vi "Setup Timer Parameters.vi"(7 "Timer Notifier":refnum<notifier>, 8 "error in (no error)":errorcluster, 9 "Count":i32, 10 "Period":i32, 11 "Timer On":bool) -> (0 "error out":errorcluster)   [LabVIEW 2015, in "Tool Module.lvlib"]
uses:
  Tool Module.lvlib
  Support/Timer Setup Params Typedef.ctl
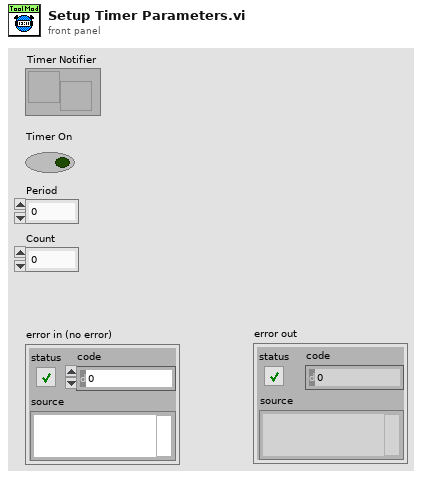
[diagram p1: front panel]
types:
  T1 = typedef "Tool Module.lvlib/Timer Setup Params Typedef.ctl" = cluster{"Timer On":bool, "Period":i32, "Count":i32}
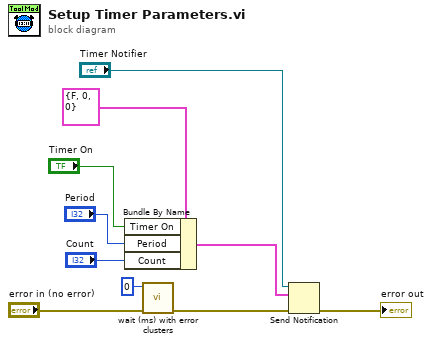
[diagram p0: block diagram]
diagram:
  n1 = Bundle By Name(cluster=T1 {"Timer On"=FALSE, "Period"=0, "Count"=0} ("_Timer Setup Params Typedef"), "Timer On"="Timer On", "Period"="Period", "Count"="Count") -> (w6:T1)
  n2 = call "wait (ms) with error clusters.vi"("error in (no error)"="error in (no error)", "milliseconds to wait"=u32 0) -> ("error out"=w2:errorcluster)  [unwired: 9 in]
  n3 = Send Notification(notification=w6, notifier="Timer Notifier", error in (no error)=w2) -> (error out=→"error out":errorcluster)  [unwired: 1 out]
